vi "Update Values.vi"(8 "error in (no error)":errorcluster, 11 "TelemetryDebug in":refnum<class "TelemetryDebug.lvclass">) -> (0 "error out":errorcluster, 3 "TelemetryDebug out":refnum<class "TelemetryDebug.lvclass">)   [LabVIEW 2020, in "VectoTools.lvlib" / "TelemetryDebug.lvclass"]
uses:
  TelemetryDebug.lvclass
  Tree Entry.ctl
  TelemetryDebug.lvclass/TelemetryDebug.ctl
  Vecto/GroupAbstract/GroupAbstract.lvclass/GroupAbstract.ctl
  Vecto/GroupAbstract/GroupAbstract.lvclass
  Vecto/NodeDiscovery/NodeDiscovery.lvclass
  Vecto/ChannelService/ChannelService.lvclass
  Vecto/Group Config/Group Config.lvclass
  Vecto/Channel Config/Channel Config.lvclass
panel:
  in  "Numeric":dbl format="%<%Y-%m-%dT%H:%M:%S%3u\n>T"
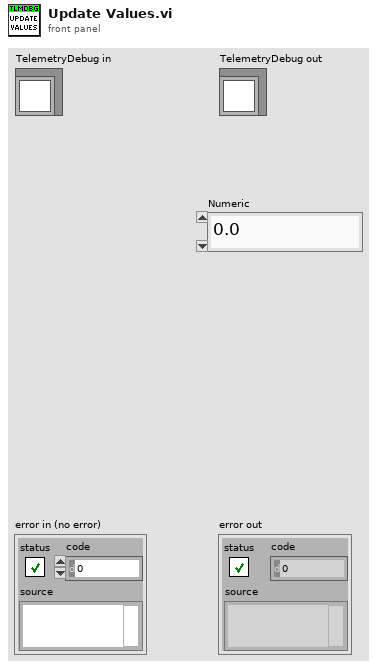
[diagram p1: front panel]
types:
  T1 = typedef "VectoTools.lvlib/TelemetryDebug.lvclass/Tree Entry.ctl" = cluster{"Hierarchy":string[], "Name":string, "Columns":string[]}
  T2 = typedef "Discovery.lvlib/Data.ctl" = cluster{"node_id":u32, "name":string, "ip":u32, "status":string, "services":T3[], "node_types":string[], "system":string, "cluster":string, "app_version":string, "cfg_version":string}
  T3 = typedef "Service.lvlib/Data.ctl" = cluster{"type":T4, "port":i32}
  T4 = typedef "ServiceType.lvlib/Enumeration.ctl" = enum16{"SERVICETYPE_UNKNOWN", "SERVICETYPE_TCPSERVER", "SERVICETYPE_HTTPSERVER"}
  T5 = typedef "LVNodeAndColumnTypeDef.ctl" = cluster{"Node":string, "Column":i32}
  T6 = typedef "Vecto.lvlib/Group Info.ctl" = cluster{"System":string, "Cluster":string, "Node":string, "Task":string, "Name":string}
  T7 = typedef "Vecto.lvlib/Channel Info.ctl" = cluster{"Name":string, "Group":string, "Owning Node":string, "Owning Task":string, "Resource":string}
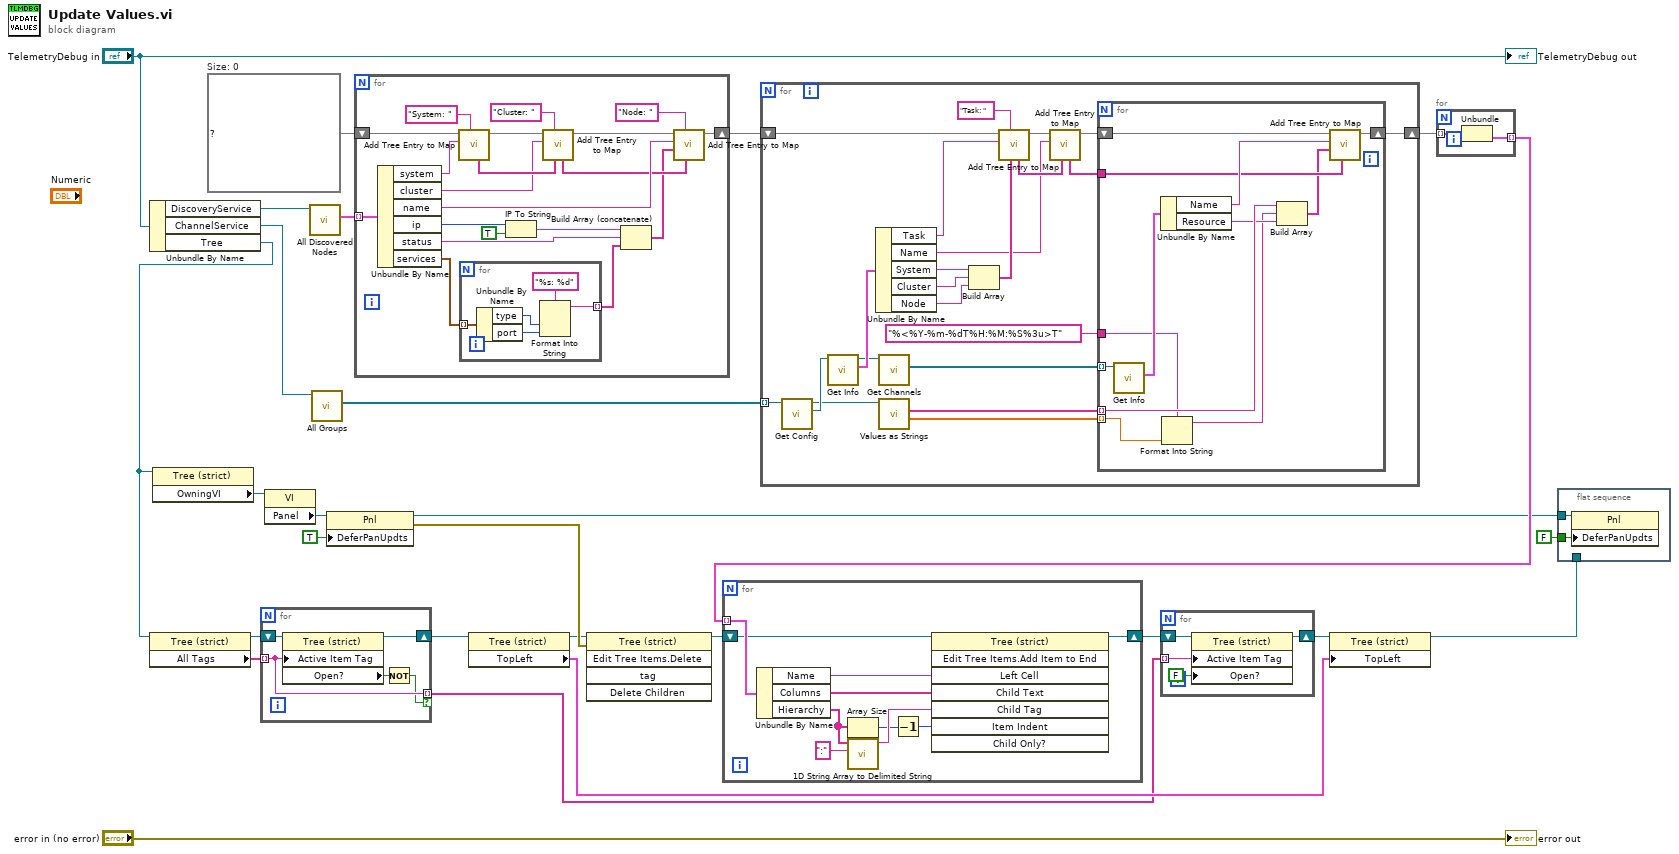
[diagram p0: block diagram]
diagram:
  w22 = map{string[], T1} {}  # Size: 0
  n1 = Unbundle By Name("TelemetryDebug in") -> ("DiscoveryService"=w24:refnum<class "NodeDiscovery.lvclass">, "ChannelService"=w14:refnum<class "ChannelService.lvclass">, "Tree"=w1:refnum<vi>)
  n2 = property class="Tree (strict)"(reference=w1) -> (reference out=w7:refnum<vi>, "All Tags"=w8:string[])  [unwired: 1 in, 1 out]
  n3 = property class="Tree (strict)"(reference=w1) -> ("OwningVI"=w19:refnum<vi>)  [unwired: 1 in, 2 out]
  n4 = for {
    tunnel: w8 -> [w30] mode=indexing
    shift-right: [w28] -> w6
    shift-left: w7 -> [w32]
    tunnel: [w30] -> w5 mode=indexing if=w29
    n5 = property class="Tree (strict)"(reference=w32, "Active Item Tag"=w30) -> (reference out=w28:refnum<vi>, "Open?"=w31:bool)  [unwired: 1 in, 1 out]
    n6 = Not(x=w31) -> (.not. x?=w29:bool)
  }
  n7 = property class="VI"(reference=w19) -> ("Panel"=w18:refnum<vi>)  [unwired: 1 in, 2 out]
  n8 = call "All Discovered Nodes.vi"("DiscoveryService in"=w24) -> ("Nodes"=w23:T2[])  [unwired: 8 in, 2 out]
  n9 = call "All Groups.vi"("ChannelService in"=w14) -> ("Groups"=w11:refnum<class "GroupAbstract.lvclass">[])  [unwired: 8 in, 2 out]
  n10 = property class="Pnl"(reference=w18, "DeferPanUpdts"=TRUE ("Defer Panel Updates")) -> (reference out=w15:refnum<vi>, error out=w27:errorcluster)  [unwired: 1 in]
  n11 = for {
    tunnel: w23 -> [w52] mode=indexing
    shift-right: [w43] -> w13
    shift-left: w22 -> [w51]
    n12 = Unbundle By Name(w52) -> ("system"=w50:string, "cluster"=w47:string, "name"=w45:string, "ip"=w42:u32, "status"=w38:string, "services"=w40:T3[])
    n13 = call "Add Tree Entry to Map.vi"("Name Prefix (none)"="System: ", "Name"=w50, "Map in"=w51) -> ("Map"=w48:map{string[], T1}, "Hierarchy"=w49:string[])  [unwired: 7 in]
    n14 = for {
      tunnel: w40 -> [w57] mode=indexing
      tunnel: [w53] -> w37 mode=indexing
      n15 = Unbundle By Name(w57) -> ("type"=w55:T4, "port"=w54:i32)
      n16 = Format Into String(format string="%s: %d", w55, w54) -> (resulting string=w53:string)  [unwired: 2 in, 1 out]
    }
    n17 = IP To String(1:TRUE ("dot notation? (F)"), 2:w42) -> (0:w39:string)
    n18 = call "Add Tree Entry to Map.vi"("Parent (None)"=w49, "Name Prefix (none)"="Cluster: ", "Name"=w47, "Map in"=w48) -> ("Map"=w46:map{string[], T1}, "Hierarchy"=w44:string[])  [unwired: 6 in]
    n19 = Build Array (concatenate)(w39, w38, w37) -> (w36:string[])
    n20 = call "Add Tree Entry to Map.vi"("Parent (None)"=w44, "Name Prefix (none)"="Node: ", "Columns"=w36, "Name"=w45, "Map in"=w46) -> ("Map"=w43:map{string[], T1})  [unwired: 5 in, 1 out]
  }
  n21 = property class="Tree (strict)"(reference=w6) -> (reference out=w10:refnum<vi>, "TopLeft"=w9:T5)  [unwired: 1 in, 1 out]
  n22 = invoke class="Tree (strict)" method="Edit Tree Items.Delete"(reference=w10, error in=w27) -> (reference out=w20:refnum<vi>)  [unwired: 3 in, 4 out]
  n23 = for {
    shift-right: [w66] -> w12
    shift-left: w13 -> [w79]
    tunnel: w11 -> [w78] mode=indexing
    n24 = call "Get Config.vi"("GroupAbstract in"=w78) -> ("Config"=w77:refnum<class "Group Config.lvclass">, "GroupAbstract out"=w62:refnum<class "GroupAbstract.lvclass">)  [unwired: 8 in, 1 out]
    n25 = call "Get Info.vi"("Group Config in"=w77) -> ("Info"=w76:T6, "Group Config out"=w64:refnum<class "Group Config.lvclass">)  [unwired: 8 in, 1 out]
    n26 = Unbundle By Name(w76) -> ("Task"=w71:string, "Name"=w68:string, "System"=w75:string, "Cluster"=w74:string, "Node"=w73:string)
    n27 = call "Get Channels.vi"("Group Config in"=w64) -> ("Channels"=w63:refnum<class "Channel Config.lvclass">[])  [unwired: 8 in, 2 out]
    n28 = call "Values as Strings.vi"("GroupAbstract in"=w62) -> ("Timestamps"=w59:dbl[], "Value Strings"=w61:string[])  [unwired: 7 in, 2 out]
    n29 = Build Array(w75, w74, w73) -> (w72:string[])
    n30 = call "Add Tree Entry to Map.vi"("Parent (None)"=w72, "Name Prefix (none)"="Task: ", "Name"=w71, "Map in"=w79) -> ("Map"=w70:map{string[], T1}, "Hierarchy"=w69:string[])  [unwired: 6 in]
    n31 = call "Add Tree Entry to Map.vi"("Parent (None)"=w69, "Name"=w68, "Map in"=w70) -> ("Map"=w67:map{string[], T1}, "Hierarchy"=w65:string[])  [unwired: 7 in]
    n32 = for {
      shift-right: [w88] -> w66
      shift-left: w67 -> [w89]
      tunnel: w65 -> [w90]
      tunnel: w61 -> [w84] mode=indexing
      tunnel: w63 -> [w86] mode=indexing
      tunnel: w59 -> [w81] mode=indexing
      tunnel: "%<%Y-%m-%dT%H:%M:%S%3u>T" ("format string") -> [w82]
      n33 = call "Get Info.vi"("Channel Config in"=w86) -> ("Info"=w85:T7)  [unwired: 8 in, 2 out]
      n34 = Unbundle By Name(w85) -> ("Name"=w91:string, "Resource"=w83:string)
      n35 = Format Into String(format string=w82, w81) -> (resulting string=w80:string)  [unwired: 2 in, 1 out]
      n36 = Build Array(w84, w80, w83) -> (w87:string[])
      n37 = call "Add Tree Entry to Map.vi"("Parent (None)"=w90, "Columns"=w87, "Name"=w91, "Map in"=w89) -> ("Map"=w88:map{string[], T1})  [unwired: 6 in, 1 out]
    }
  }
  n38 = for {
    tunnel: w12 -> [w93] mode=indexing
    tunnel: [w92] -> w21 mode=indexing
    n39 = Unbundle(w93) -> ("Tree Entry"=w92:T1)  [unwired: 1 out]
  }
  n40 = for {
    tunnel: w21 -> [w103] mode=indexing
    shift-right: [w94] -> w2
    shift-left: w20 -> [w102]
    n41 = Unbundle By Name(w103) -> ("Name"=w101:string, "Columns"=w100:string[], "Hierarchy"=w97:string[])
    n42 = Array Size(array=w97) -> (size(s)=w96:i32)
    n43 = call <vilib>:"1D String Array to Delimited String.vi"("delimiter"=":", "string array"=w97) -> ("delimited string"=w98:string)  [unwired: 9 in]
    n44 = Decrement(x=w96) -> (x-1=w95:i32)
    n45 = invoke class="Tree (strict)" method="Edit Tree Items.Add Item to End"(reference=w102, "Left Cell"=w101, "Child Text"=w100, "Child Tag"=w98, "Item Indent"=w95) -> (reference out=w94:refnum<vi>)  [unwired: 3 in, 7 out]
  }
  n46 = for {
    shift-right: [w106] -> w4
    shift-left: w2 -> [w107]
    tunnel: w5 -> [w104] mode=indexing
    n47 = property class="Tree (strict)"(reference=w107, "Active Item Tag"=w104, "Open?"=FALSE ("Active Item:Open?")) -> (reference out=w106:refnum<vi>)  [unwired: 1 in, 1 out]
  }
  n48 = property class="Tree (strict)"(reference=w4, "TopLeft"=w9) -> (reference out=w3:refnum<vi>)  [unwired: 1 in, 1 out]
  n49 = flat-sequence {
    tunnel: FALSE ("Defer Panel Updates") -> [w109]
    tunnel: w15 -> [w108]
    tunnel: w3 -> [_]
    frame #0 {
      n50 = property class="Pnl"(reference=w108, "DeferPanUpdts"=w109) -> ()  [unwired: 1 in, 2 out]
    }
  }
  "error out" <- "error in (no error)"
  "TelemetryDebug out" <- "TelemetryDebug in"
